vi "Labview Gyro Test.vi"() -> ()   [LabVIEW 2016]
doc: "This example performs writes and reads on a serial port, as directed by the user. You can press the Write and Read buttons, and change the Read Count, while the example is running.\n\nThe parameters set for the serial port must match the parameters of the connected instrument or device. In this example, the Read Count parameter specifies the number of bytes that the serial port reads. If there were more bytes at the port than the specified number, those bytes would not be read. If there were less bytes at the port than the specified number, you would receive a timeout error.\n\nThis example expands upon the flow control options for XON and XOFF, allowing the user to choose those control characters. Also, the user can enable or disable a termination character. Some devices require a termination character in order to identify the end of command strings. Some devices send a termination character to signify the end of data to be read. This example shows how you can end the Read operation once a termination character is detected in the buffer and/or append a termination character at the end of the Write data."
uses:
  <vilib>/Instr/_visa.llb/VISA Configure Serial Port (Instr).vi
  <vilib>/picture/3D Picture Control/Object/Create Object (name).vi
  <vilib>/picture/3D Picture Control/NI_3D Picture Control.lvlib
panel:
  in  "Big slope":dbl=12.0
  in  "Log recording":bool
  out "Numeric Control":i32
  out "Flag":bool
  in  "?":bool
  in  "?":bool
  in  "?":bool
  in  "?":bool
  in  "?":bool
  in  "?":bool
  out "?":string
  in  "Level 6":dbl=3.3 min=0.0 max=3.3
  in  "Level 5":dbl=3.0 min=0.0 max=3.3
  in  "Level 4":dbl=2.4 min=0.0 max=3.3
  in  "Level 3":dbl=1.8 min=0.0 max=3.3
  in  "Level 2":dbl=1.2 min=0.0 max=3.3
  in  "Level 1":dbl=0.6 min=0.0 max=3.3
  out "Force":string
  out "3D Picture":refnum<vi>(3d-picture)
  in  "Connect":bool
  out "Pitch":string
  in  "Small slope":dbl=5.0
  in  "Downhill":dbl=-5.0
  out "?":string
  out "Roll":string
  in  "Read Count":u32=1000
  in  "Select COM port":refnum<visa-resource-name>="COM1"
  out "?":dbl(graph)
  out "?":dbl(graph)
  out "?":dbl(graph)
  out "Yaw":string
  out "?":dbl(graph)
  # "Save&Load\nConfiguration"
  # "The Max. Range of Levels"
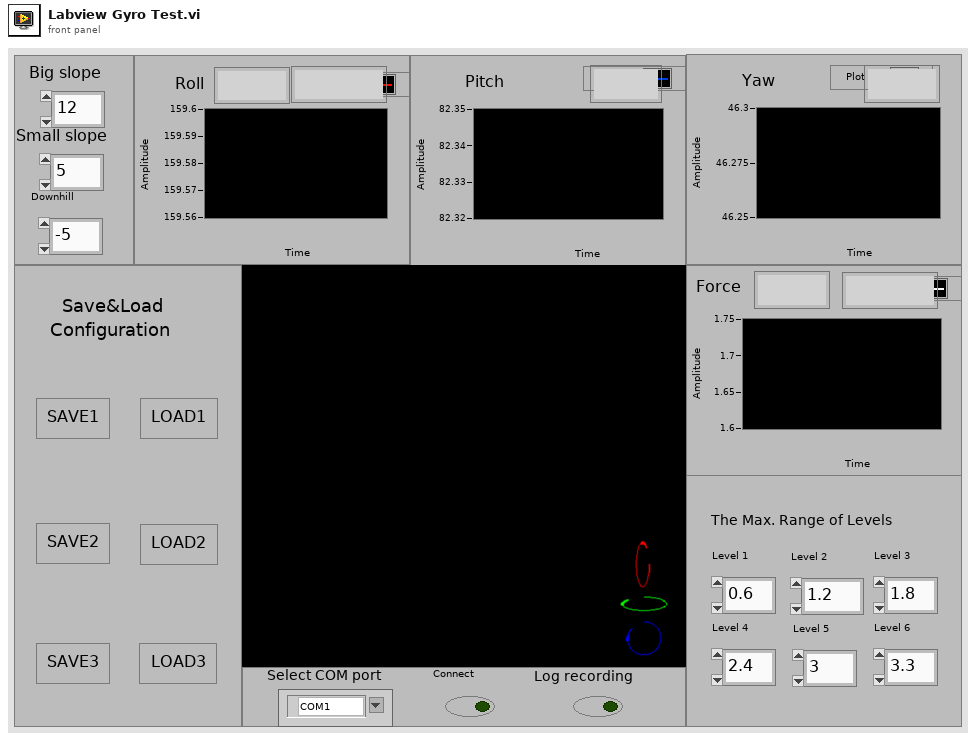
[diagram p1: front panel]
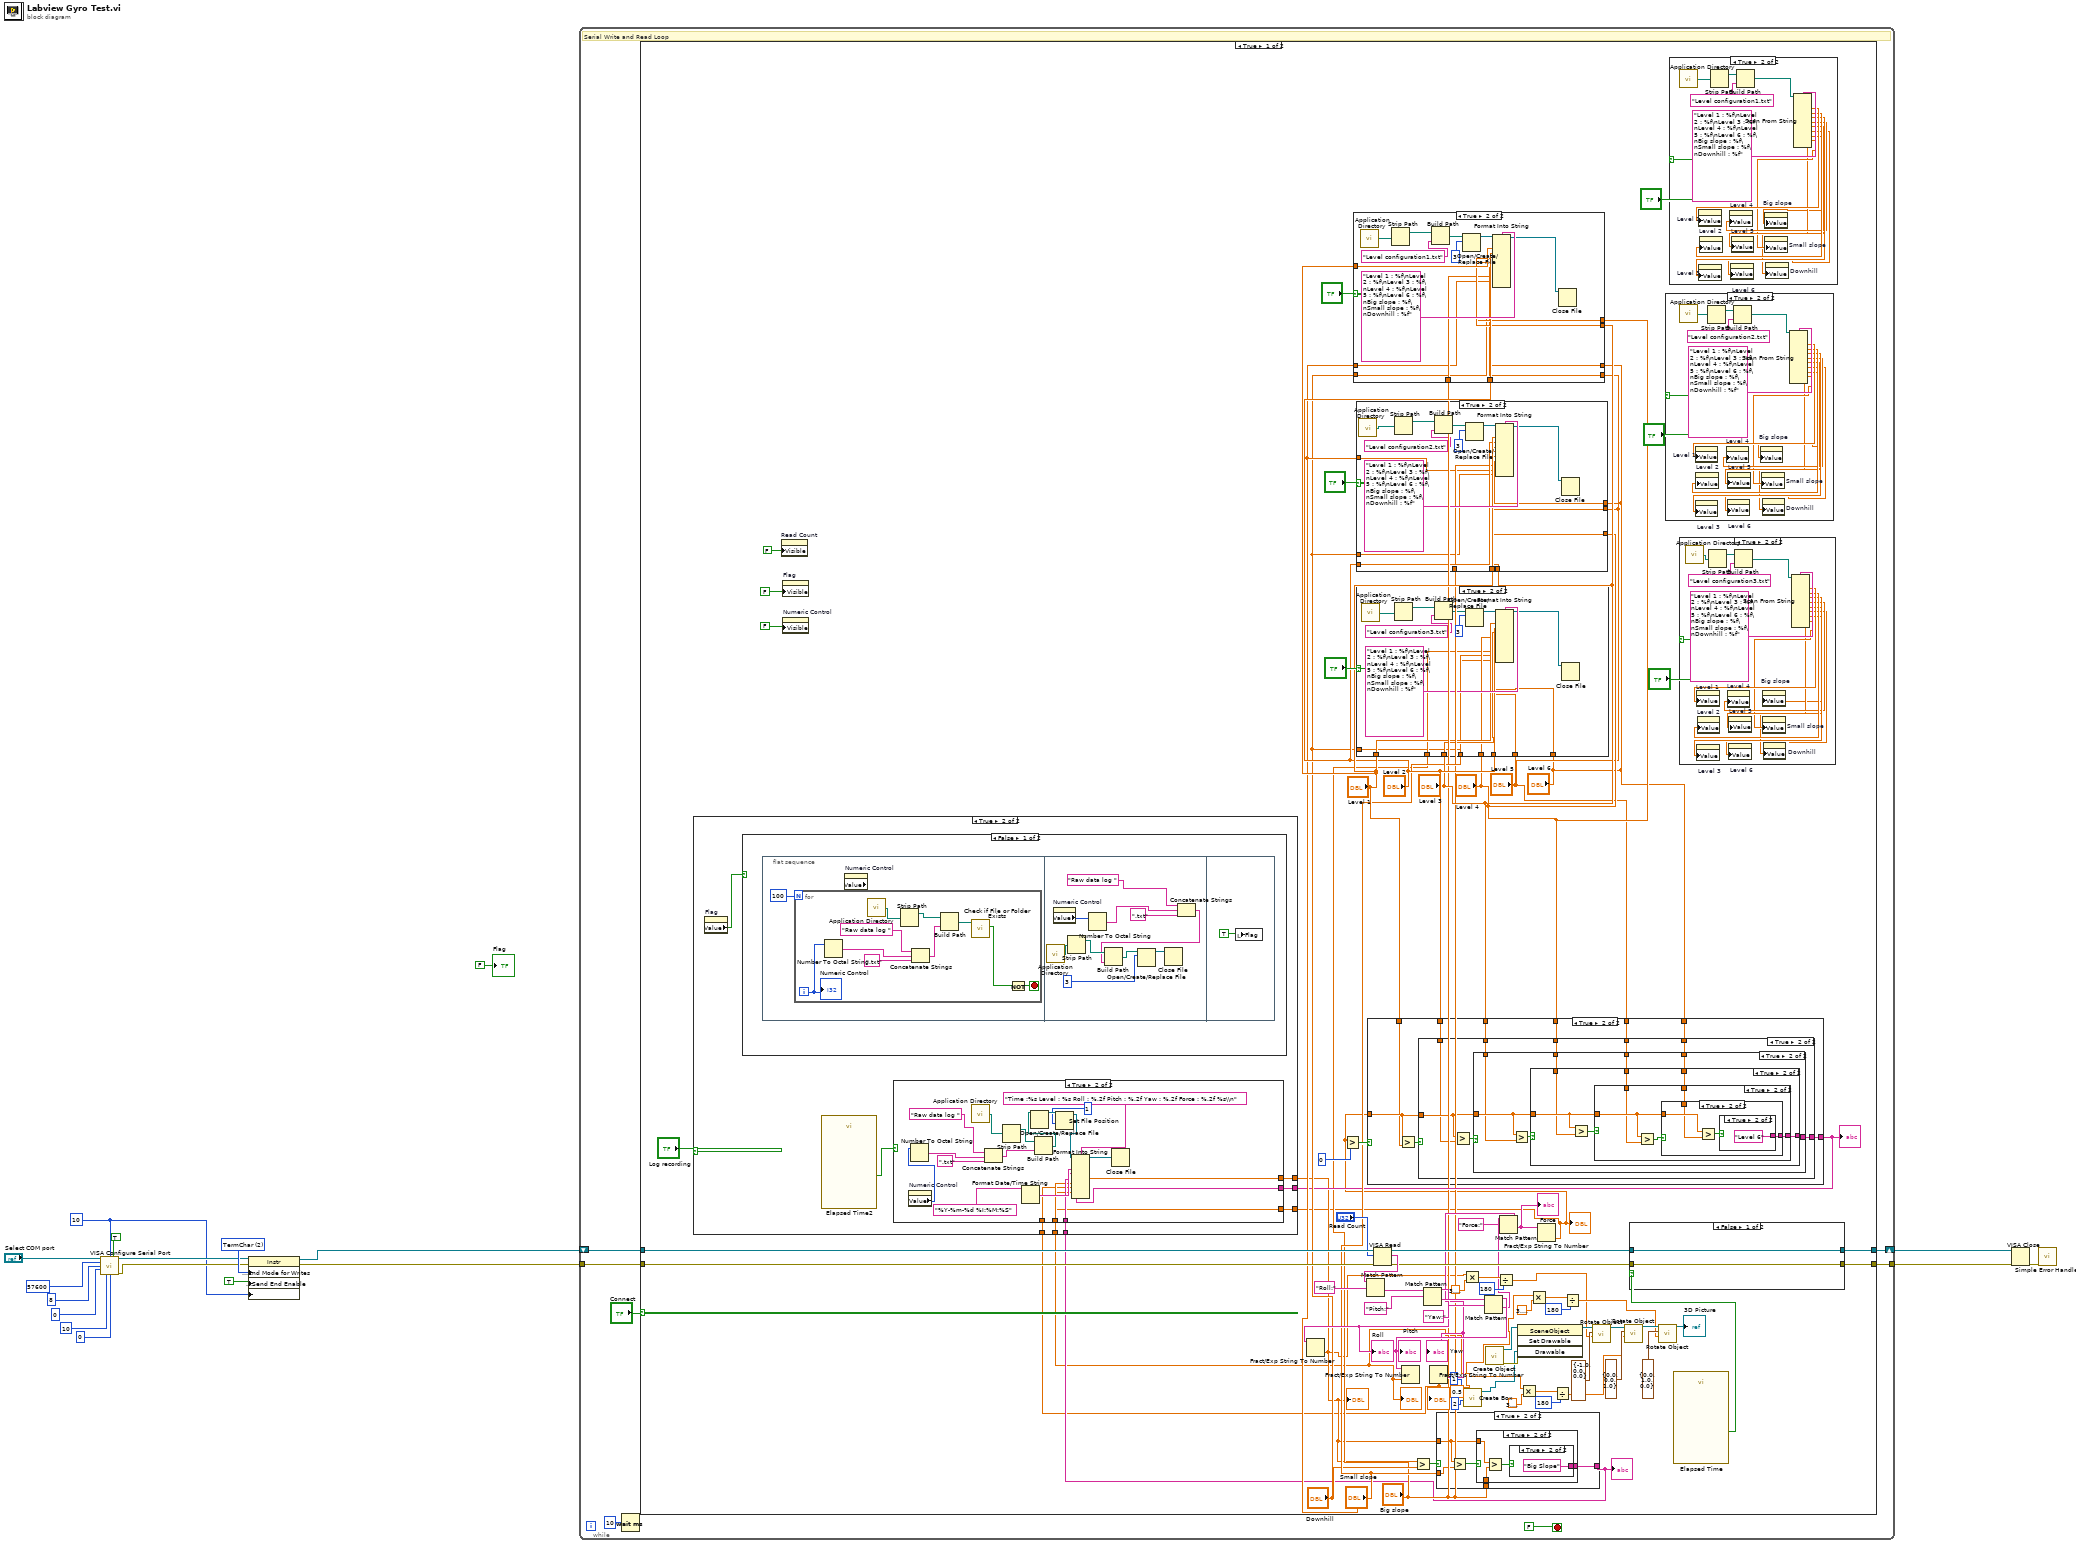
[diagram p0: block diagram]
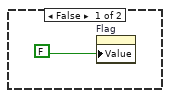
[diagram p2: hidden frame]
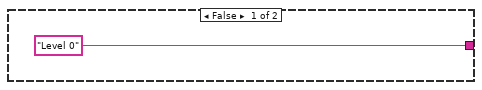
[diagram p11: hidden frame]
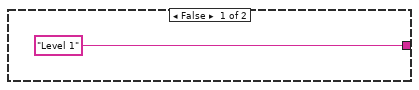
[diagram p12: hidden frame]
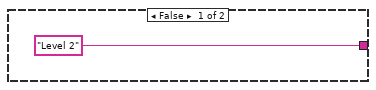
[diagram p13: hidden frame]
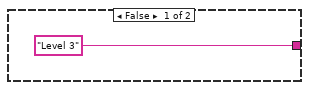
[diagram p14: hidden frame]
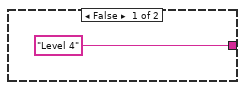
[diagram p15: hidden frame]
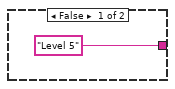
[diagram p16: hidden frame]
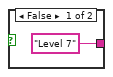
[diagram p17: hidden frame]
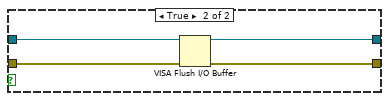
[diagram p18: hidden frame]
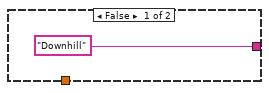
[diagram p19: hidden frame]
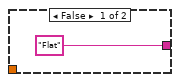
[diagram p20: hidden frame]
diagram:
  w7 = u16 2 items=["None", "LastBit", "TermChar", "Break"] ("Serial Settings:Serial End Mode for Writes")
  w3 = 10
  n1 = call-poly "VISA Configure Serial Port"("VISA resource name"="Select COM port", "termination char\n(0xA = '\\n' = LF)"=w3, "Enable Termination\nChar (T)"=TRUE, "baud rate (9600)"=57600, "data bits (8)"=8, "parity (0:none)"=0, "stop bits (10: 1 bit)"=10, "flow control (0:none)"=0) -> ("VISA resource name out"=w6:refnum<visa-resource-name>, "error out"=w4:errorcluster)  [unwired: 2 in, 4 out]
  n2 = property class="Instr"(reference=w6, error in=w4, "Serial Settings:End Mode for Writes"=w7, "Message Based Settings:Send End Enable"=TRUE, "Message Based Settings:Termination Character"=w3) -> (reference out=w5:refnum<visa-resource-name>, error out=w2:errorcluster)
  n3 = while {
    shift-right: [w25] -> w15
    shift-left: w5 -> [w21]
    tunnel: w2 -> [w20]
    tunnel: [w23] -> w16
    stop <- FALSE stop-if-true
    # "Serial Write and Read Loop"
    n4 = Wait (ms)(milliseconds to wait=u32 10) -> ()  [unwired: 1 out]
    n5 = case shown="True" "Connect" {
      tunnel: [w64 w312] -> w25
      tunnel: w21 -> [w98 w313]
      tunnel: [w61 w310] -> w23
      tunnel: w20 -> [w97 w311]
      frame True {
        n6 = property on="Read Count" class="DigNum (strict)"("Visible"=FALSE) -> ()  [unwired: 2 in, 2 out]
        n7 = property on="Flag" class="Bool (strict)"("Visible"=FALSE) -> ()  [unwired: 2 in, 2 out]
        n8 = property on="Numeric Control" class="DigNum (strict)"("Visible"=FALSE) -> ()  [unwired: 2 in, 2 out]
        n9 = case shown="True" "?" {
          tunnel: "Level 1" -> [_ w202]
          tunnel: "Level 2" -> [_ w201]
          tunnel: "Level 3" -> [_ w200]
          tunnel: "Level 4" -> [_ w199]
          tunnel: "Level 5" -> [_ w198]
          tunnel: "Level 6" -> [_ w197]
          tunnel: "Big slope" -> [_ w196]
          tunnel: "Small slope" -> [_ w195]
          tunnel: "Downhill" -> [_ w194]
          frame False {
          }
          frame True {
            n10 = call <vilib>:"Application Directory.vi"() -> ("Application Directory"=w193:path)
            n11 = Strip Path(path=w193) -> (stripped path=w209:path)  [unwired: 1 out]
            n12 = Build Path(base path=w209, name or relative path="Level configuration1.txt") -> (appended path=w207:path)
            n13 = Open/Create/Replace File(file path (use dialog)=w207, operation (0:open)=3) -> (refnum out=w205:refnum<file>)  [unwired: 4 in, 2 out]
            n14 = Format Into String(format string="Level 1 : %f\nLevel 2 : %f\nLevel 3 : %f\nLevel 4 : %f\nLevel 5 : %f\nLevel 6 : %f\nBig slope : %f\nSmall slope : %f\nDownhill : %f", initial string=w205, w202, w201, w200, w199, w198, w197, w196, w195, w194) -> (resulting string=w203:refnum<file>)  [unwired: 1 in, 1 out]
            n15 = Close File(refnum=w203) -> ()  [unwired: 1 in, 2 out]
          }
        }
        n16 = case shown="True" "?" {
          tunnel: "Level 1" -> [_ w219]
          tunnel: "Level 2" -> [_ w218]
          tunnel: "Level 3" -> [_ w217]
          tunnel: "Level 4" -> [_ w216]
          tunnel: "Level 5" -> [_ w215]
          tunnel: "Level 6" -> [_ w214]
          tunnel: "Big slope" -> [_ w213]
          tunnel: "Small slope" -> [_ w212]
          tunnel: "Downhill" -> [_ w211]
          frame False {
          }
          frame True {
            n17 = call <vilib>:"Application Directory.vi"() -> ("Application Directory"=w210:path)
            n18 = Strip Path(path=w210) -> (stripped path=w226:path)  [unwired: 1 out]
            n19 = Build Path(base path=w226, name or relative path="Level configuration2.txt") -> (appended path=w224:path)
            n20 = Open/Create/Replace File(file path (use dialog)=w224, operation (0:open)=3) -> (refnum out=w222:refnum<file>)  [unwired: 4 in, 2 out]
            n21 = Format Into String(format string="Level 1 : %f\nLevel 2 : %f\nLevel 3 : %f\nLevel 4 : %f\nLevel 5 : %f\nLevel 6 : %f\nBig slope : %f\nSmall slope : %f\nDownhill : %f", initial string=w222, w219, w218, w217, w216, w215, w214, w213, w212, w211) -> (resulting string=w220:refnum<file>)  [unwired: 1 in, 1 out]
            n22 = Close File(refnum=w220) -> ()  [unwired: 1 in, 2 out]
          }
        }
        n23 = case shown="True" "?" {
          tunnel: "Level 1" -> [_ w236]
          tunnel: "Level 2" -> [_ w235]
          tunnel: "Level 3" -> [_ w234]
          tunnel: "Level 4" -> [_ w233]
          tunnel: "Level 5" -> [_ w232]
          tunnel: "Level 6" -> [_ w231]
          tunnel: "Big slope" -> [_ w230]
          tunnel: "Small slope" -> [_ w229]
          tunnel: "Downhill" -> [_ w228]
          frame False {
          }
          frame True {
            n24 = call <vilib>:"Application Directory.vi"() -> ("Application Directory"=w227:path)
            n25 = Strip Path(path=w227) -> (stripped path=w243:path)  [unwired: 1 out]
            n26 = Build Path(base path=w243, name or relative path="Level configuration3.txt") -> (appended path=w241:path)
            n27 = Open/Create/Replace File(file path (use dialog)=w241, operation (0:open)=3) -> (refnum out=w239:refnum<file>)  [unwired: 4 in, 2 out]
            n28 = Format Into String(format string="Level 1 : %f\nLevel 2 : %f\nLevel 3 : %f\nLevel 4 : %f\nLevel 5 : %f\nLevel 6 : %f\nBig slope : %f\nSmall slope : %f\nDownhill : %f", initial string=w239, w236, w235, w234, w233, w232, w231, w230, w229, w228) -> (resulting string=w237:refnum<file>)  [unwired: 1 in, 1 out]
            n29 = Close File(refnum=w237) -> ()  [unwired: 1 in, 2 out]
          }
        }
        n30 = VISA Read(VISA resource name=w98, byte count="Read Count", error in (no error)=w97) -> (VISA resource name out=w63:refnum<visa-resource-name>, read buffer=w88:string, error out=w62:errorcluster)  [unwired: 1 out]
        n31 = Match Pattern(string=w88, regular expression="Roll:") -> (after substring=w94:string)  [unwired: 1 in, 3 out]
        n32 = Match Pattern(string=w94, regular expression="Pitch:") -> (before substring=w89:string, after substring=w93:string)  [unwired: 1 in, 2 out]
        "Roll" <- w89
        n33 = Fract/Exp String To Number(string=w89) -> (number=w29:dbl)  [unwired: 3 in, 1 out]
        "?" <- w29
        n34 = Greater?(x=w29, y="Downhill") -> (0:w92:bool)
        n35 = case shown="True" w92 {
          tunnel: ["Downhill" w301] -> w30
          tunnel: w29 -> [_ w300]
          tunnel: "Small slope" -> [_ w299]
          tunnel: "Big slope" -> [_ w298]
          frame False {
          }
          frame True {
            n36 = Greater?(x=w300, y=w299) -> (0:w302:bool)
            n37 = case shown="True" w302 {
              tunnel: ["Flat" w307] -> w301
              tunnel: w300 -> [_ w305]
              tunnel: w298 -> [_ w304]
              frame False {
              }
              frame True {
                n38 = Greater?(x=w305, y=w304) -> (0:w306:bool)
                n39 = case shown="True" w306 {
                  tunnel: ["Small Slope" "Big Slope"] -> w307
                  frame False {
                  }
                  frame True {
                  }
                }
              }
            }
          }
        }
        "?" <- w30
        n40 = Multiply(x=w29, y=3.141592653589793) -> (x*y=w67:dbl)
        n41 = call <vilib>:"Create Box.vi"("Length Z"=2, "Length Y"=0.5, "Length X"=1) -> ("New Box Refnum"=w54:refnum<vi>)  [unwired: 7 in, 1 out]
        n42 = Match Pattern(string=w93, regular expression="Yaw:") -> (before substring=w87:string, after substring=w60:string)  [unwired: 1 in, 2 out]
        "Pitch" <- w87
        n43 = Fract/Exp String To Number(string=w87) -> (number=w28:dbl)  [unwired: 3 in, 1 out]
        "?" <- w28
        n44 = call-poly <vilib>:"Create Object.vi"() -> ("error out"=w79:errorcluster, "Scene:New Object"=w78:refnum<vi>)  [unwired: 10 in]
        n45 = Divide(x=w67, y=180) -> (x/y=w66:dbl)
        n46 = Match Pattern(string=w60, regular expression="Force:") -> (before substring=w57:string, after substring=w58:string)  [unwired: 1 in, 2 out]
        "Yaw" <- w57
        "Force" <- w58
        n47 = Fract/Exp String To Number(string=w57) -> (number=w27:dbl)  [unwired: 3 in, 1 out]
        "?" <- w27
        n48 = invoke class="SceneObject" method="Set Drawable"(reference=w78, error in=w79, "Drawable"=w54) -> (reference out=w80:refnum<vi>)  [unwired: 1 in, 3 out]
        n49 = Multiply(x=w28, y=3.141592653589793) -> (x*y=w71:dbl)
        n50 = Multiply(x=w27, y=3.141592653589793) -> (x*y=w77:dbl)
        n51 = Fract/Exp String To Number(string=w58) -> (number=w26:dbl)  [unwired: 3 in, 1 out]
        "?" <- w26
        n52 = Greater?(x=w26, y=0) -> (0:w56:bool)
        n53 = case shown="True" w56 {
          tunnel: w26 -> [_ w252]
          tunnel: ["Level 0" w251] -> w34
          tunnel: "Level 1" -> [_ w250]
          tunnel: "Level 2" -> [_ w249]
          tunnel: "Level 3" -> [_ w248]
          tunnel: "Level 4" -> [_ w247]
          tunnel: "Level 5" -> [_ w246]
          tunnel: "Level 6" -> [_ w245]
          frame False {
          }
          frame True {
            n54 = Greater?(x=w252, y=w250) -> (0:w253:bool)
            n55 = case shown="True" w253 {
              tunnel: w252 -> [_ w261]
              tunnel: ["Level 1" w260] -> w251
              tunnel: w249 -> [_ w259]
              tunnel: w248 -> [_ w258]
              tunnel: w247 -> [_ w257]
              tunnel: w246 -> [_ w256]
              tunnel: w245 -> [_ w255]
              frame False {
              }
              frame True {
                n56 = Greater?(x=w261, y=w259) -> (0:w262:bool)
                n57 = case shown="True" w262 {
                  tunnel: w261 -> [_ w269]
                  tunnel: ["Level 2" w268] -> w260
                  tunnel: w258 -> [_ w267]
                  tunnel: w257 -> [_ w266]
                  tunnel: w256 -> [_ w265]
                  tunnel: w255 -> [_ w264]
                  frame False {
                  }
                  frame True {
                    n58 = Greater?(x=w269, y=w267) -> (0:w270:bool)
                    n59 = case shown="True" w270 {
                      tunnel: w269 -> [_ w276]
                      tunnel: ["Level 3" w275] -> w268
                      tunnel: w266 -> [_ w274]
                      tunnel: w265 -> [_ w273]
                      tunnel: w264 -> [_ w272]
                      frame False {
                      }
                      frame True {
                        n60 = Greater?(x=w276, y=w274) -> (0:w277:bool)
                        n61 = case shown="True" w277 {
                          tunnel: w276 -> [_ w282]
                          tunnel: ["Level 4" w281] -> w275
                          tunnel: w273 -> [_ w280]
                          tunnel: w272 -> [_ w279]
                          frame False {
                          }
                          frame True {
                            n62 = Greater?(x=w282, y=w280) -> (0:w283:bool)
                            n63 = case shown="True" w283 {
                              tunnel: w282 -> [_ w288]
                              tunnel: ["Level 5" w286] -> w281
                              tunnel: w279 -> [_ w285]
                              frame False {
                              }
                              frame True {
                                n64 = Greater?(x=w288, y=w285) -> (0:w287:bool)
                                n65 = case shown="True" w287 {
                                tunnel: ["Level 7" "Level 6"] -> w286
                                frame False {
                                }
                                frame True {
                                }
                                }
                              }
                            }
                          }
                        }
                      }
                    }
                  }
                }
              }
            }
          }
        }
        "?" <- w34
        n66 = case shown="True" "Log recording" {
          tunnel: w34 -> [_ w106]
          tunnel: w30 -> [_ w104]
          tunnel: w29 -> [_ w103]
          tunnel: w28 -> [_ w102]
          tunnel: w27 -> [_ w101]
          tunnel: w26 -> [_ w100]
          frame False {
            n67 = property on="Flag" class="Bool (strict)"("Value"=FALSE) -> ()  [unwired: 2 in, 2 out]
          }
          frame True {
            n68 = property on="Flag" class="Bool (strict)"() -> ("Value"=w105:bool)  [unwired: 2 in, 2 out]
            n69 = case shown="False" w105 {
              frame False {
                n70 = flat-sequence {
                  frame #0 {
                    n71 = for {
                      N: 100 -> [_]
                      i -> [w112]
                      stop <- w113 stop-if-true
                      n72 = Number To Octal String(2:w112) -> (0:w114:string)  [unwired: 1 in]
                      n73 = call <vilib>:"Application Directory.vi"() -> ("Application Directory"=w110:path)
                      n74 = Strip Path(path=w110) -> (stripped path=w109:path)  [unwired: 1 out]
                      n75 = Concatenate Strings("Raw data log ", w114, ".txt") -> (w117:string)
                      n76 = Build Path(base path=w109, name or relative path=w117) -> (appended path=w116:path)
                      n77 = call <vilib>:"Check if File or Folder Exists.vi"("path"=w116) -> ("file or folder exists?"=w111:bool)  [unwired: 8 in, 2 out]
                      n78 = Not(x=w111) -> (.not. x?=w113:bool)
                      "Numeric Control" <- w112
                    }
                    n79 = property on="Numeric Control" class="DigNum (strict)" props=["Value"]() -> ()  [unwired: 2 in, 3 out]
                  }
                  frame #1 {
                    n80 = call <vilib>:"Application Directory.vi"() -> ("Application Directory"=w120:path)
                    n81 = property on="Numeric Control" class="DigNum (strict)"() -> ("Value"=w127:i32)  [unwired: 2 in, 2 out]
                    n82 = Strip Path(path=w120) -> (stripped path=w125:path)  [unwired: 1 out]
                    n83 = Number To Octal String(2:w127) -> (0:w128:string)  [unwired: 1 in]
                    n84 = Concatenate Strings("Raw data log ", w128, ".txt") -> (w124:string)
                    n85 = Build Path(base path=w125, name or relative path=w124) -> (appended path=w123:path)
                    n86 = Open/Create/Replace File(file path (use dialog)=w123, operation (0:open)=3) -> (refnum out=w121:refnum<file>)  [unwired: 4 in, 2 out]
                    n87 = Close File(refnum=w121) -> ()  [unwired: 1 in, 2 out]
                  }
                  frame #2 {
                    n88 = local write "Flag"(TRUE) -> ()
                  }
                }
              }
              frame True {
              }
            }
            n89 = call "Elapsed Time2"() -> ("Time has Elapsed"=w107:bool)  [unwired: 12 in, 7 out]
            n90 = case shown="True" w107 {
              tunnel: w106 -> [_ w139]
              tunnel: w104 -> [_ w134]
              tunnel: w103 -> [_ w133]
              tunnel: w102 -> [_ w132]
              tunnel: w101 -> [_ w131]
              tunnel: w100 -> [_ w130]
              frame False {
              }
              frame True {
                n91 = property on="Numeric Control" class="DigNum (strict)"() -> ("Value"=w145:i32)  [unwired: 2 in, 2 out]
                n92 = Number To Octal String(2:w145) -> (0:w147:string)  [unwired: 1 in]
                n93 = call <vilib>:"Application Directory.vi"() -> ("Application Directory"=w138:path)
                n94 = Concatenate Strings("Raw data log ", w147, ".txt") -> (w144:string)
                n95 = Strip Path(path=w138) -> (stripped path=w150:path)  [unwired: 1 out]
                n96 = Format Date/Time String(time format string (%c)="%Y-%m-%d %I:%M:%S") -> (date/time string=w136:string)  [unwired: 2 in]
                n97 = Build Path(base path=w150, name or relative path=w144) -> (appended path=w142:path)
                n98 = Open/Create/Replace File(file path (use dialog)=w142) -> (refnum out=w141:refnum<file>)  [unwired: 5 in, 2 out]
                n99 = Set File Position(refnum=w141, from (0:start)=1) -> (refnum out=w143:refnum<file>)  [unwired: 2 in, 1 out]
                n100 = Format Into String(format string="Time :%s Level : %s Roll : %.2f Pitch : %.2f Yaw : %.2f Force : %.2f %s\\n", initial string=w143, w136, w134, w133, w132, w131, w130, w139) -> (resulting string=w148:refnum<file>)  [unwired: 1 in, 1 out]
                n101 = Close File(refnum=w148) -> ()  [unwired: 1 in, 2 out]
              }
            }
          }
        }
        n102 = Divide(x=w71, y=180) -> (x/y=w70:dbl)
        n103 = Divide(x=w77, y=180) -> (x/y=w74:dbl)
        n104 = call <vilib>:"Rotate Object.vi"("Angle"=w66, "Axis"=cluster{"X":sgl, "Y":sgl, "Z":sgl} {"X"=-1.0, "Y"=0.0, "Z"=0.0} ("Translation"), "Scene.Object In"=w80) -> ("Scene.Object Out"=w84:refnum<vi>)  [unwired: 7 in, 1 out]
        n105 = call <vilib>:"Rotate Object.vi"("Angle"=w70, "Axis"=cluster{"X":sgl, "Y":sgl, "Z":sgl} {"X"=0.0, "Y"=0.0, "Z"=1.0} ("Translation"), "Scene.Object In"=w84) -> ("Scene.Object Out"=w85:refnum<vi>)  [unwired: 7 in, 1 out]
        n106 = call <vilib>:"Rotate Object.vi"("Angle"=w74, "Axis"=cluster{"X":sgl, "Y":sgl, "Z":sgl} {"X"=0.0, "Y"=1.0, "Z"=0.0} ("Translation"), "Scene.Object In"=w85) -> ("Scene.Object Out"=→"3D Picture":refnum<vi>)  [unwired: 7 in, 1 out]
        n107 = case shown="True" "?" {
          frame False {
          }
          frame True {
            n108 = call <vilib>:"Application Directory.vi"() -> ("Application Directory"=w165:path)
            n109 = Strip Path(path=w165) -> (stripped path=w178:path)  [unwired: 1 out]
            n110 = Build Path(base path=w178, name or relative path="Level configuration2.txt") -> (appended path=w176:path)
            n111 = Scan From String("Level 1 : %f\nLevel 2 : %f\nLevel 3 : %f\nLevel 4 : %f\nLevel 5 : %f\nLevel 6 : %f\nBig slope : %f\nSmall slope : %f\nDownhill : %f", w176) -> (output 1=w174:dbl, output 2=w173:dbl, output 3=w172:dbl, output 4=w171:dbl, output 5=w170:dbl, output 6=w169:dbl, output 7=w166:dbl, output 8=w168:dbl, output 9=w167:dbl)  [unwired: 10 in, 2 out]
            n112 = property on="Level 1" class="DigNum (strict)"("Value"=w174) -> ()  [unwired: 2 in, 2 out]
            n113 = property on="Level 3" class="DigNum (strict)"("Value"=w172) -> ()  [unwired: 2 in, 2 out]
            n114 = property on="Level 2" class="DigNum (strict)"("Value"=w173) -> ()  [unwired: 2 in, 2 out]
            n115 = property on="Level 4" class="DigNum (strict)"("Value"=w171) -> ()  [unwired: 2 in, 2 out]
            n116 = property on="Level 6" class="DigNum (strict)"("Value"=w169) -> ()  [unwired: 2 in, 2 out]
            n117 = property on="Level 5" class="DigNum (strict)"("Value"=w170) -> ()  [unwired: 2 in, 2 out]
            n118 = property on="Big slope" class="DigNum (strict)"("Value"=w166) -> ()  [unwired: 2 in, 2 out]
            n119 = property on="Small slope" class="DigNum (strict)"("Value"=w168) -> ()  [unwired: 2 in, 2 out]
            n120 = property on="Downhill" class="DigNum (strict)"("Value"=w167) -> ()  [unwired: 2 in, 2 out]
          }
        }
        n121 = case shown="True" "?" {
          frame False {
          }
          frame True {
            n122 = call <vilib>:"Application Directory.vi"() -> ("Application Directory"=w151:path)
            n123 = Strip Path(path=w151) -> (stripped path=w164:path)  [unwired: 1 out]
            n124 = Build Path(base path=w164, name or relative path="Level configuration1.txt") -> (appended path=w162:path)
            n125 = Scan From String("Level 1 : %f\nLevel 2 : %f\nLevel 3 : %f\nLevel 4 : %f\nLevel 5 : %f\nLevel 6 : %f\nBig slope : %f\nSmall slope : %f\nDownhill : %f", w162) -> (output 1=w160:dbl, output 2=w159:dbl, output 3=w158:dbl, output 4=w157:dbl, output 5=w156:dbl, output 6=w155:dbl, output 7=w152:dbl, output 8=w154:dbl, output 9=w153:dbl)  [unwired: 10 in, 2 out]
            n126 = property on="Level 1" class="DigNum (strict)"("Value"=w160) -> ()  [unwired: 2 in, 2 out]
            n127 = property on="Level 3" class="DigNum (strict)"("Value"=w158) -> ()  [unwired: 2 in, 2 out]
            n128 = property on="Level 2" class="DigNum (strict)"("Value"=w159) -> ()  [unwired: 2 in, 2 out]
            n129 = property on="Level 4" class="DigNum (strict)"("Value"=w157) -> ()  [unwired: 2 in, 2 out]
            n130 = property on="Level 6" class="DigNum (strict)"("Value"=w155) -> ()  [unwired: 2 in, 2 out]
            n131 = property on="Level 5" class="DigNum (strict)"("Value"=w156) -> ()  [unwired: 2 in, 2 out]
            n132 = property on="Big slope" class="DigNum (strict)"("Value"=w152) -> ()  [unwired: 2 in, 2 out]
            n133 = property on="Small slope" class="DigNum (strict)"("Value"=w154) -> ()  [unwired: 2 in, 2 out]
            n134 = property on="Downhill" class="DigNum (strict)"("Value"=w153) -> ()  [unwired: 2 in, 2 out]
          }
        }
        n135 = call "Elapsed Time"() -> ("Time has Elapsed"=w65:bool)  [unwired: 12 in, 7 out]
        n136 = case shown="False" w65 {
          tunnel: [w292 w296] -> w64
          tunnel: w63 -> [w292 w295]
          tunnel: w62 -> [w291 w294]
          tunnel: [w291 w293] -> w61
          frame False {
          }
          frame True {
            n137 = VISA Flush I/O Buffer(VISA resource name=w295, error in (no error)=w294) -> (VISA resource name out=w296:refnum<visa-resource-name>, error out=w293:errorcluster)  [unwired: 1 in]
          }
        }
        n138 = case shown="True" "?" {
          frame False {
          }
          frame True {
            n139 = call <vilib>:"Application Directory.vi"() -> ("Application Directory"=w179:path)
            n140 = Strip Path(path=w179) -> (stripped path=w192:path)  [unwired: 1 out]
            n141 = Build Path(base path=w192, name or relative path="Level configuration3.txt") -> (appended path=w190:path)
            n142 = Scan From String("Level 1 : %f\nLevel 2 : %f\nLevel 3 : %f\nLevel 4 : %f\nLevel 5 : %f\nLevel 6 : %f\nBig slope : %f\nSmall slope : %f\nDownhill : %f", w190) -> (output 1=w188:dbl, output 2=w187:dbl, output 3=w186:dbl, output 4=w185:dbl, output 5=w184:dbl, output 6=w183:dbl, output 7=w180:dbl, output 8=w182:dbl, output 9=w181:dbl)  [unwired: 10 in, 2 out]
            n143 = property on="Level 1" class="DigNum (strict)"("Value"=w188) -> ()  [unwired: 2 in, 2 out]
            n144 = property on="Level 3" class="DigNum (strict)"("Value"=w186) -> ()  [unwired: 2 in, 2 out]
            n145 = property on="Level 2" class="DigNum (strict)"("Value"=w187) -> ()  [unwired: 2 in, 2 out]
            n146 = property on="Level 4" class="DigNum (strict)"("Value"=w185) -> ()  [unwired: 2 in, 2 out]
            n147 = property on="Level 6" class="DigNum (strict)"("Value"=w183) -> ()  [unwired: 2 in, 2 out]
            n148 = property on="Level 5" class="DigNum (strict)"("Value"=w184) -> ()  [unwired: 2 in, 2 out]
            n149 = property on="Big slope" class="DigNum (strict)"("Value"=w180) -> ()  [unwired: 2 in, 2 out]
            n150 = property on="Small slope" class="DigNum (strict)"("Value"=w182) -> ()  [unwired: 2 in, 2 out]
            n151 = property on="Downhill" class="DigNum (strict)"("Value"=w181) -> ()  [unwired: 2 in, 2 out]
          }
        }
      }
      frame False {
        n152 = VISA Flush I/O Buffer(VISA resource name=w313, error in (no error)=w311) -> (VISA resource name out=w312:refnum<visa-resource-name>, error out=w310:errorcluster)  [unwired: 1 in]
      }
    }
  }
  n153 = VISA Close(VISA resource name=w15, error in (no error)=w16) -> (error out=w17:errorcluster)
  n154 = call <vilib>:"Simple Error Handler.vi"("error in (no error)"=w17) -> ()  [unwired: 1 in, 8 out]
  "Flag" <- FALSE
